vi "Read Store Value.vi"(11 "Store Value in":refnum<class "Store Value Msg.lvclass">) -> (1 "Value":string, 2 "Key":string, 3 "Store Value out":refnum<class "Store Value Msg.lvclass">)   [LabVIEW 2015, in "IED Actor.lvlib" / "Store Value Msg.lvclass"]
uses:
  Store Value Msg.lvclass
  Store Value Msg.lvclass/Store Value Msg.ctl
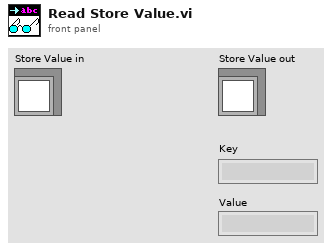
[diagram p1: front panel]
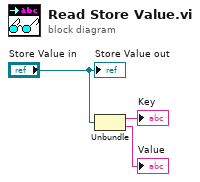
[diagram p0: block diagram]
diagram:
  n1 = Unbundle("Store Value in") -> (→"Key":string, →"Value":string)
  "Store Value out" <- "Store Value in"
